vi "ErrorLog_GetErrors.vi"(8 "error in (no error)":errorcluster, 11 "reference in":refnum<class "ErrorLog.lvclass">) -> (0 "error out":errorcluster, 1 "Errors since last call":string, 2 "New Errors":bool, 3 "reference out":refnum<class "ErrorLog.lvclass">, 4 "Errors since last clear":string, 5 "Uncleared Errors":bool)   [LabVIEW 2014, in "ErrorLog.lvclass"]
uses:
  ErrorLog.lvclass
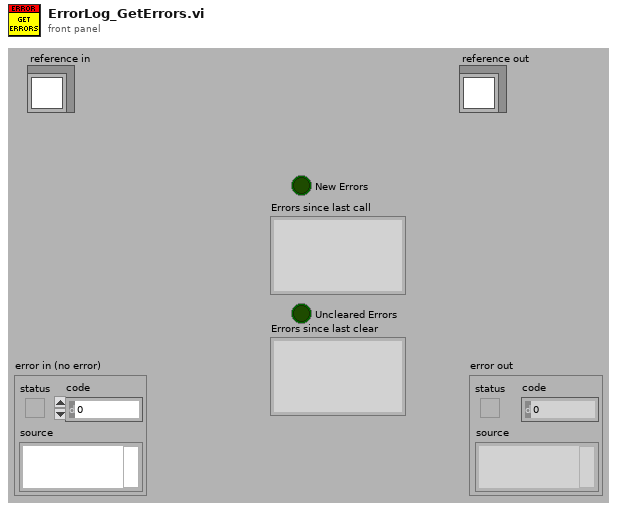
[diagram p1: front panel]
types:
  T1 = typedef "ErrorLog.lvclass/ObjectAttributes.ctl" = cluster{"ErrorFile":path, "Supress Consecutive Duplicates":bool, "Errors":string, "Quit":bool, "Errors since last call":string, "Last Recorded Error":string, "ErrorPath":path, "PossiblePaths":path[], "BaseFileName":string, "Max Log Files":i32, "ErrorFile Index":i32, "Max File Size":i64}
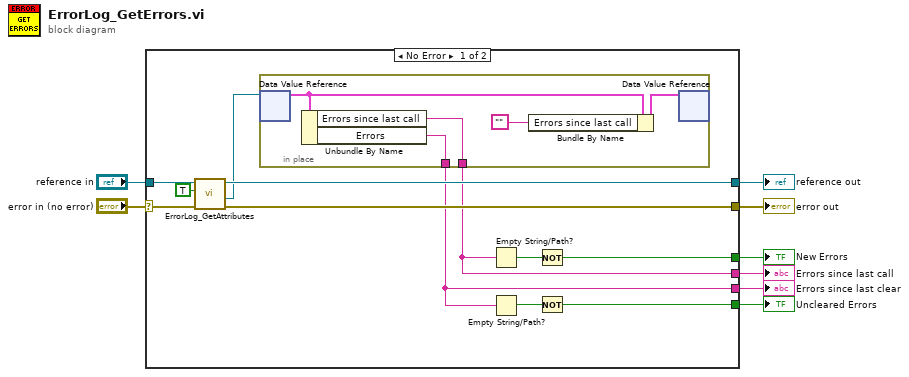
[diagram p0: block diagram]
diagram:
  n1 = case shown="No Error" "error in (no error)" {
    selector: "error in (no error)" -> [w20 w27]
    tunnel: [w18 w27] -> w7
    tunnel: [w13 w26] -> w5
    tunnel: "reference in" -> [w19 w26]
    tunnel: [w10 _] -> w4
    tunnel: [w9 _] -> w3
    tunnel: [w15 _] -> w2
    tunnel: [w14 _] -> w1
    frame No Error {
      n2 = call "ErrorLog_GetAttributes.vi"("error in (no error)"=w20, "OnlyGetDvrReference(False)"=TRUE, "reference in"=w19) -> ("error out"=w18:errorcluster, "DataRef"=w11:refnum<data-value>, "reference out"=w13:refnum<class "ErrorLog.lvclass">)  [unwired: 5 in, 1 out]
      n3 = in-place {
        in-place-border: [w25] -> w10
        in-place-border: [w24] -> w9
        n4 = in-place-dvr #1(w11) -> (w23:T1)  [unwired: 1 out]
        n5 = Unbundle By Name(w23) -> ("Errors since last call"=w25:string, "Errors"=w24:string)
        n6 = Bundle By Name(cluster=w23, "Errors since last call"="") -> (w22:T1)
        n7 = in-place-dvr #1(w22) -> ()  [unwired: 2 out]
      }
      n8 = Empty String/Path?(string/path=w10) -> (empty?=w17:bool)
      n9 = Empty String/Path?(string/path=w9) -> (empty?=w16:bool)
      n10 = Not(x=w17) -> (.not. x?=w14:bool)
      n11 = Not(x=w16) -> (.not. x?=w15:bool)
    }
    frame Error {
    }
  }
  "error out" <- w7
  "reference out" <- w5
  "Errors since last call" <- w4
  "New Errors" <- w1
  "Errors since last clear" <- w3
  "Uncleared Errors" <- w2
